vi "Monitorserie_labview.vi"() -> ()   [LabVIEW 2020]
uses:
  <vilib>/Instr/_visa.llb/VISA Configure Serial Port (Instr).vi
  <vilib>/regexp/Match Regular Expression.xnode
panel:
  out "Respuesta":string
  out "O2 %":dbl(slide) scale=-10.0..10.0
  out "O2 V":dbl(slide) scale=0.0..1.0
  out "O2 %":dbl
  out "O2 V":dbl
  out "kPa":dbl
  out "kPa":dbl(knob) scale=0.0..750.0
  in  "Server Closed":string="The server VI closed the connection."
  in  "baud rate (115200)":u32=9600
  in  "Flow control":u16(ring) items=["None"=0, "XON/XOFF"=1, "RTS/CTS"=2, "DTR/DSR"=4]
  in  "Stop bits":u16(ring)=10 items=["1.0"=10, "1.5"=15, "2.0"=20]
  in  "Paridad":u16(ring) items=["None", "Odd", "Even", "Mark", "Space"]
  in  "Data bits     :":u16=8 min=5 max=8 step=1
  in  "VISA resource : name:":refnum<visa-resource-name>="COM1"
  in  "stop":bool
  out "Read buffer":string
  # "Configuracion Parámetros"
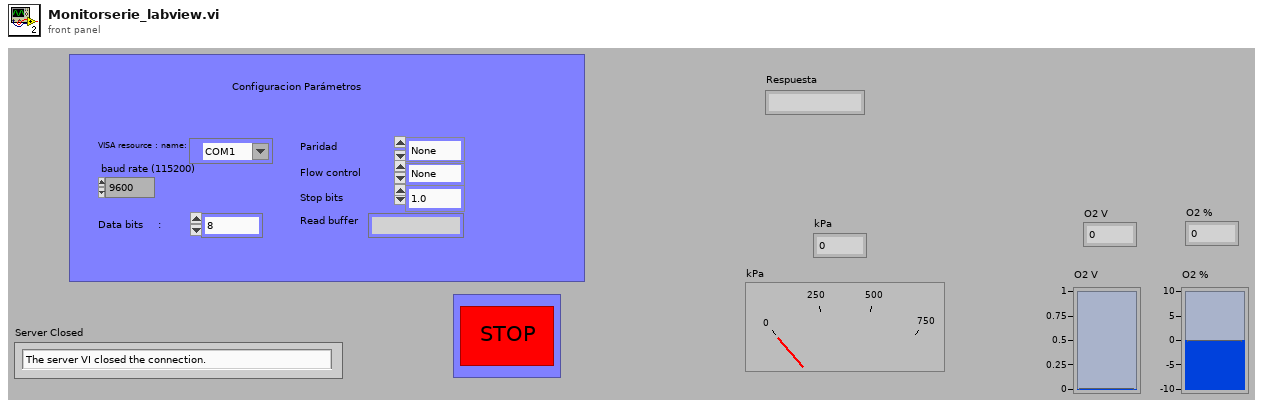
[diagram p1: front panel]
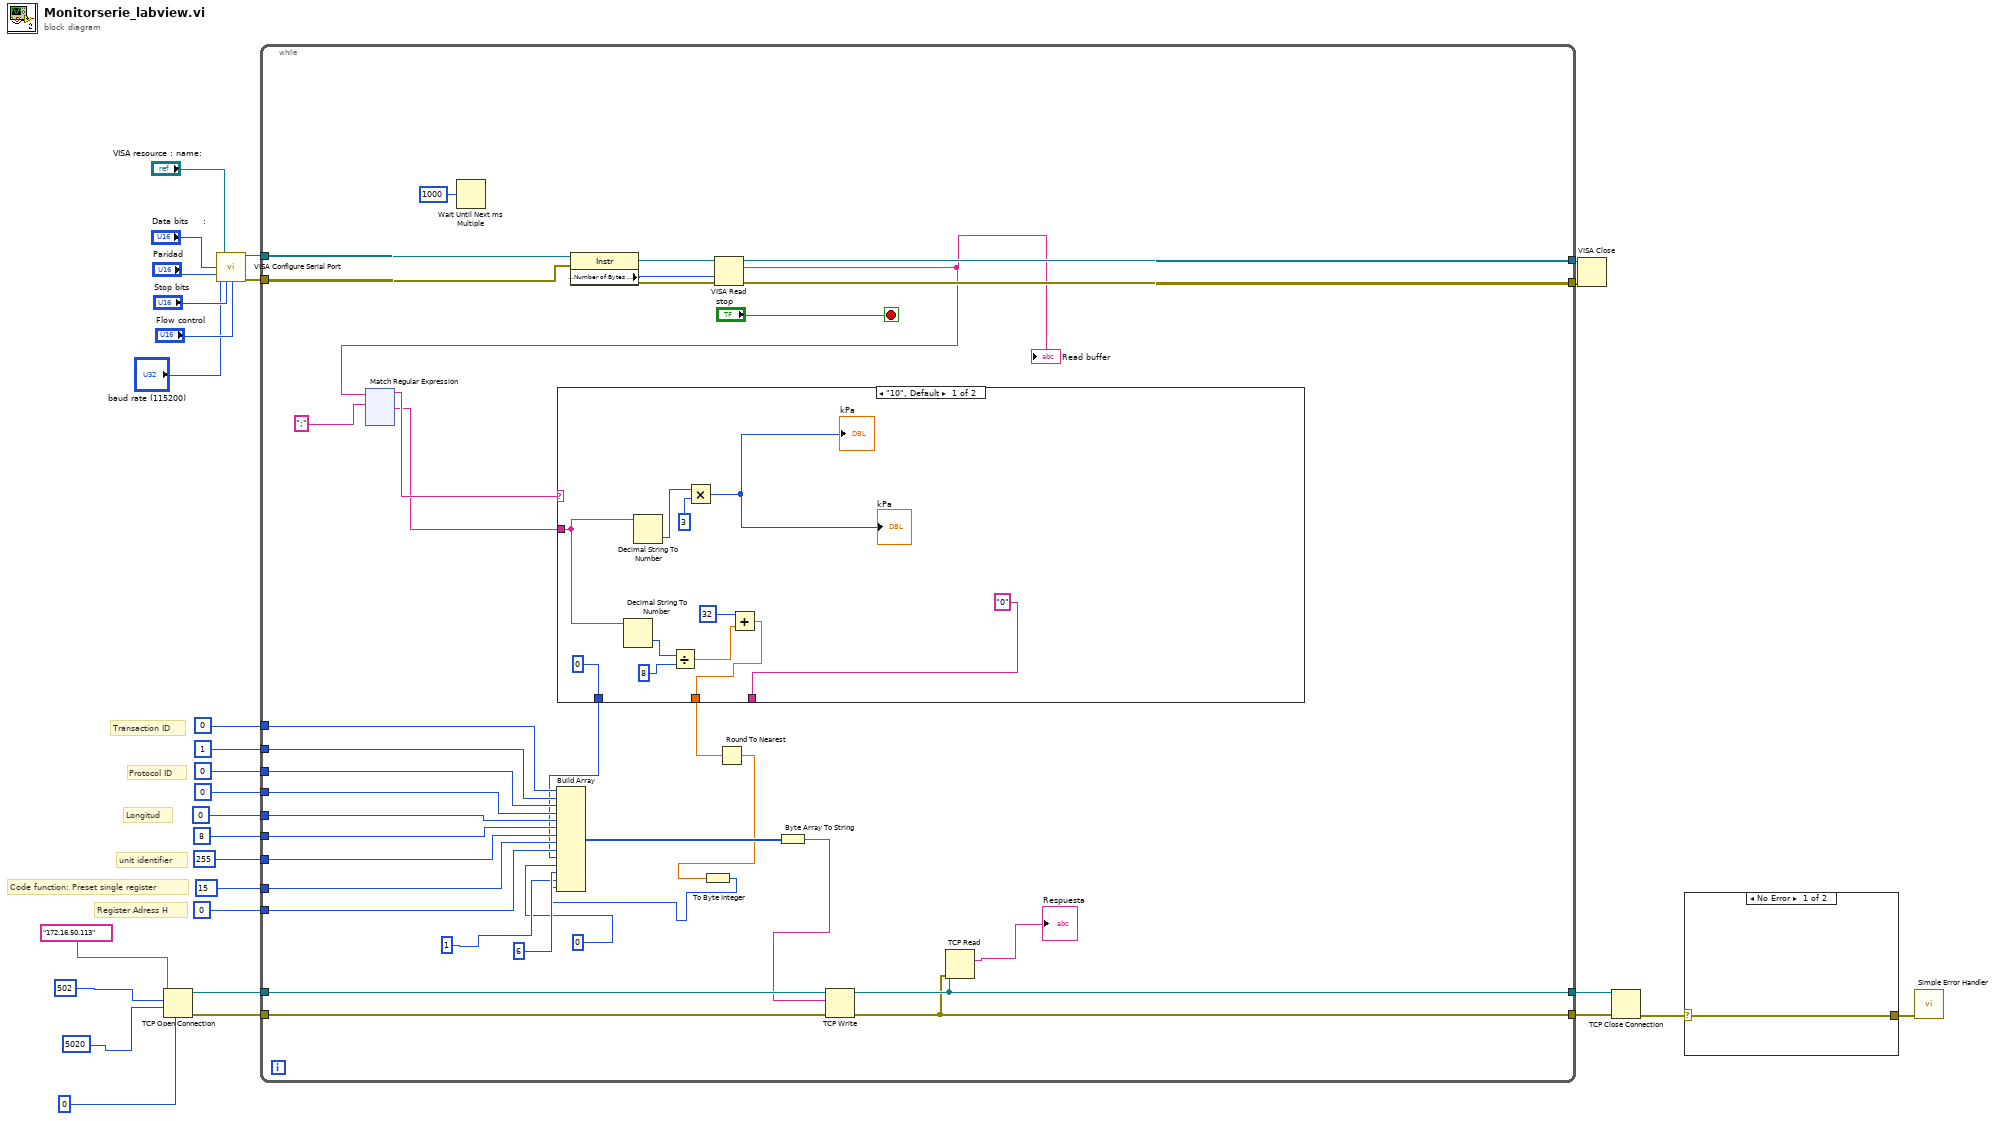
[diagram p0: block diagram]
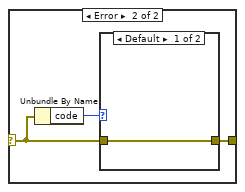
[diagram p2: hidden frame]
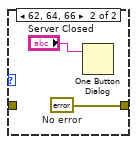
[diagram p3: hidden frame]
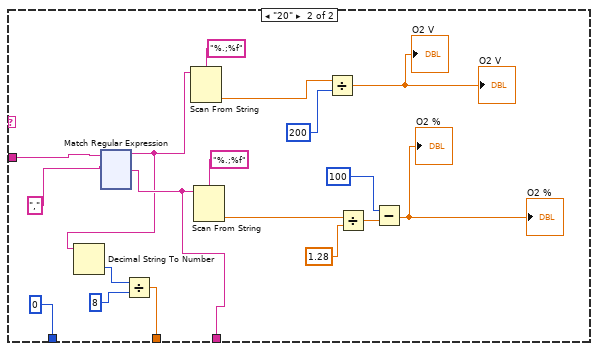
[diagram p4: hidden frame]
diagram:
  # "Register Adress H"
  # "Longitud"
  # "Transaction ID"
  # "Protocol ID"
  # "unit identifier"
  # "Code function: Preset single register"
  n1 = TCP Open Connection(address="172.16.50.113", remote port or service name=502, timeout ms (60000)=5020, local port=0) -> (connection ID=w6:refnum<k5>, error out=w5:errorcluster)  [unwired: 1 in]
  n2 = call-poly "VISA Configure Serial Port"("VISA resource name"="VISA resource : name:", "baud rate (9600)"="baud rate (115200)", "data bits (8)"="Data bits     :", "parity (0:none)"="Paridad", "stop bits (10: 1 bit)"="Stop bits", "flow control (0:none)"="Flow control") -> ("VISA resource name out"=w24:refnum<visa-resource-name>, "error out"=w23:errorcluster)  [unwired: 8 in]
  n3 = while {
    tunnel: w24 -> [w64]
    tunnel: w23 -> [w63]
    tunnel: [w59] -> w22
    tunnel: [w58] -> w21
    tunnel: u8 0 -> [w42]
    tunnel: u8 1 -> [w56]
    tunnel: u8 0 -> [w55]
    tunnel: u8 0 -> [w54]
    tunnel: u8 0 -> [w53]
    tunnel: u8 8 -> [w52]
    tunnel: u8 255 -> [w51]
    tunnel: u8 15 -> [w50]
    tunnel: u8 0 -> [w49]
    tunnel: w6 -> [w47]
    tunnel: w5 -> [w48]
    tunnel: [w38] -> w1
    tunnel: [w37] -> w2
    stop <- "stop" stop-if-true
    n4 = Wait Until Next ms Multiple(millisecond multiple=u32 1000) -> ()  [unwired: 1 out]
    n5 = property class="Instr"(reference=w64, error in=w63) -> (reference out=w65:refnum<visa-resource-name>, error out=w62:errorcluster, "Serial Settings:Number of Bytes at Serial Port"=w57:u32)
    n6 = VISA Read(VISA resource name=w65, byte count=w57, error in (no error)=w62) -> (VISA resource name out=w58:refnum<visa-resource-name>, read buffer=w45:string, error out=w59:errorcluster)  [unwired: 1 out]
    "Read buffer" <- w45
    n7 = xnode "Match Regular Expression"("input string"=w45, "regular expression"=";") -> ("before match"=w44:string, "after match"=w43:string)  [unwired: 4 in, 3 out]
    n8 = case shown="\"10\", Default" w44 {
      tunnel: w43 -> [w187 w208]
      tunnel: ["0" w196] -> _
      tunnel: [w181 w192] -> w33
      tunnel: [0 0] -> w31
      frame "10", Default {
        n9 = Decimal String To Number(string=w187) -> (number=w185:i32)  [unwired: 2 in, 1 out]
        n10 = Decimal String To Number(string=w187) -> (number=w190:i32)  [unwired: 2 in, 1 out]
        n11 = Divide(x=w185, y=8) -> (x/y=w182:dbl)
        n12 = Multiply(x=w190, y=3) -> (x*y=→"kPa" →"kPa":i32)
        n13 = Add(x=32, y=w182) -> (x+y=w181:dbl)
      }
      frame "20" {
        n14 = xnode "Match Regular Expression"("input string"=w208, "regular expression"=",") -> ("before match"=w193:string, "after match"=w196:string)  [unwired: 4 in, 3 out]
        n15 = Decimal String To Number(string=w193) -> (number=w195:i32)  [unwired: 2 in, 1 out]
        n16 = Divide(x=w195, y=8) -> (x/y=w192:dbl)
        n17 = Scan From String(format string="%.;%f", input string=w193) -> (output 1=w197:dbl)  [unwired: 3 in, 3 out]
        n18 = Scan From String(format string="%.;%f", input string=w196) -> (output 1=w201:dbl)  [unwired: 3 in, 3 out]
        n19 = Divide(x=w197, y=200) -> (x/y=→"O2 V" →"O2 V":dbl)
        n20 = Divide(x=w201, y=1.28) -> (x/y=w200:dbl)
        n21 = Subtract(x=100, y=w200) -> (x-y=→"O2 %" →"O2 %":dbl)
      }
    }
    n22 = Round To Nearest(number=w33) -> (nearest integer value=w34:dbl)
    n23 = To Byte Integer(number=w34) -> (8bit integer=w30:i8)
    n24 = Build Array(w42, w56, w55, w54, w53, w52, w51, w50, w49, w31, 0, 6, 1, w30) -> (w40:i32[])
    n25 = Byte Array To String(unsigned byte array=w40) -> (string=w39:string)
    n26 = TCP Write(connection ID=w47, data in=w39, error in (no error)=w48) -> (connection ID out=w38:refnum<k5>, error out=w37:errorcluster)  [unwired: 1 in, 1 out]
    n27 = TCP Read(connection ID=w38, error in (no error)=w37) -> (data out=→"Respuesta":string)  [unwired: 3 in, 2 out]
  }
  n28 = VISA Close(VISA resource name=w21, error in (no error)=w22) -> ()  [unwired: 1 out]
  n29 = TCP Close Connection(connection ID=w1, error in (no error)=w2) -> (error out=w3:errorcluster)  [unwired: 1 in, 1 out]
  n30 = case shown="No Error" w3 {
    selector: w3 -> [w323 w325]
    tunnel: [w323 w324] -> w4
    frame No Error {
    }
    frame Error {
      n31 = Unbundle By Name(w325) -> ("code"=w326:i32)
      n32 = case shown="Default" w326 {
        tunnel: w325 -> [w327 _]
        tunnel: [w327 w329] -> w324
        frame Default {
        }
        frame 62, 64, 66 {
          w329 = errorcluster {"status"=FALSE, "code"=0, "source"=""}  # No error
          n33 = One Button Dialog(message="Server Closed") -> ()  [unwired: 1 in, 1 out]
        }
      }
    }
  }
  n34 = call <vilib>:"Simple Error Handler.vi"("error in (no error)"=w4) -> ()  [unwired: 4 in, 5 out]
